vi "Get_freq.vi"(8 "error in (no error)":errorcluster, 11 "RF in":refnum<class "Store.lvclass">) -> (0 "error out":errorcluster, 3 "RF out":refnum<class "Store.lvclass">)   [LabVIEW 2019]
uses:
  Store.lvclass
panel:
  out "Bit rate":dbl=32.0
  out "Carrier":dbl=13560.0
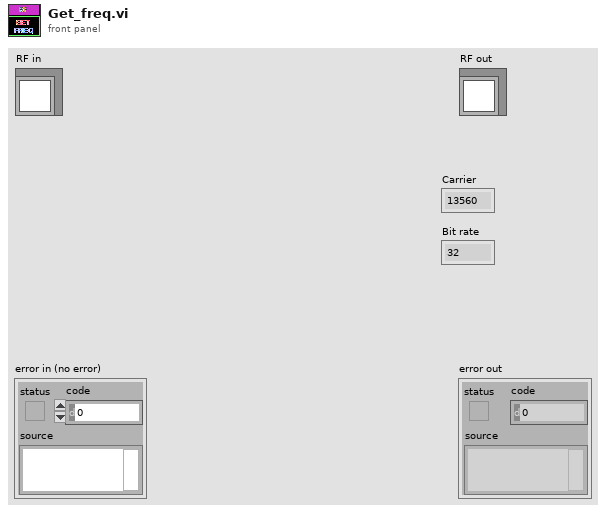
[diagram p1: front panel]
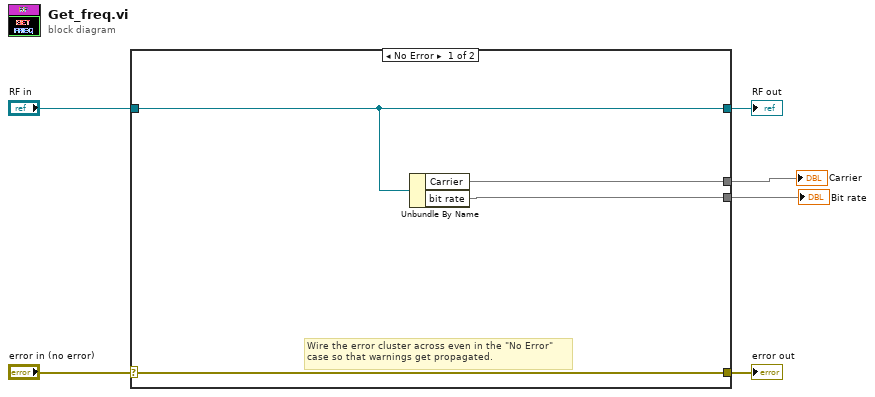
[diagram p0: block diagram]
diagram:
  n1 = case shown="No Error" "error in (no error)" {
    selector: "error in (no error)" -> [w10 w12]
    tunnel: [w10 w12] -> w5
    tunnel: [w9 w11] -> w3
    tunnel: "RF in" -> [w9 w11]
    tunnel: [w8 _] -> w2
    tunnel: [w7 _] -> w1
    frame No Error {
      # "Wire the error cluster across even in the \"No Error\"\ncase so that warnings get propagated."
      n2 = Unbundle By Name(w9) -> ("Carrier"=w8, "bit rate"=w7)
    }
    frame Error {
    }
  }
  "error out" <- w5
  "RF out" <- w3
  "Carrier" <- w2
  "Bit rate" <- w1
